vi "SS2 Live_Update Settings & Control.vi"(8 "Error In":errorcluster, 9 "Value":variant, 10 "Sender":string="SS2 DAQ", 11 "CtlRef":refnum<vi>) -> (0 "Error Out":errorcluster, 2 "Control Label":string)   [LabVIEW 2019]
uses:
  SS2 Live_Settings Event.ctl
  SS2 Live_Settings Window Messages.ctl
  Notebook/Notebook.lvlib
  Rich Text Box/Rich Text Box.lvlib
  SS2 Live_Settings List.ctl
  Variant/Variant to Data/Variant to Data.lvlib
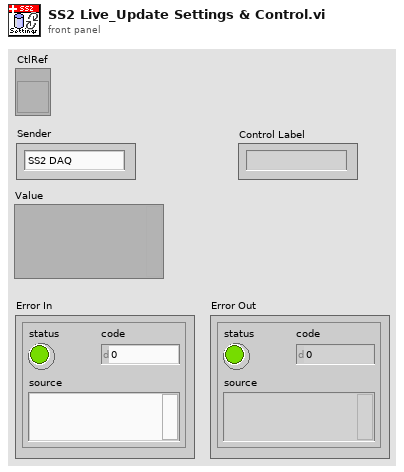
[diagram p1: front panel]
types:
  T1 = typedef "SS2 Live_Settings Event.ctl" = cluster{"Settings Message":T2, "Sender":string, "Control Label":string, "Data":variant}
  T2 = typedef "SS2 Live_Settings Window Messages.ctl" = enum16{"Idle", "Subscribe", "Unsubscribe", "Refresh Parameter", "Refresh All Parameters", "Quit"}
  T3 = typedef "SS2 Live_Settings List.ctl" = enum16{"FPGA:Bitfile Path", "FPGA:Bitfile Version", "Acquisition Parameters:SS2 DAQ Parameters", "Acquisition Parameters:Gate Configuration Array", "Acquisition Parameters:Buffer Size (# Gates)", "File Information:File Information", "File Information:# Datasets in Series", "Image Parameters:Image ROI Information", "Image Parameters:Image Binning Options", "UI Parameters:Histogram Bins Number"}
  T4 = typedef "Rich Text Box.lvlib/Text Formatting.ctl" = cluster{"Font":string, "Text Color":T5, "Text Background Color":T5, "Text Style":enum16{"Regular", "Bold", "Italic", "Underline", "Strikeout"}, "Font Size (Points)":dbl, "Text Alignment":i32}
  T5 = typedef "Rich Text Box.lvlib/Text Colors.ctl" = enum16{"Unchanged", "Black", "Blue", "Gray", "Green", "Red", "White"}
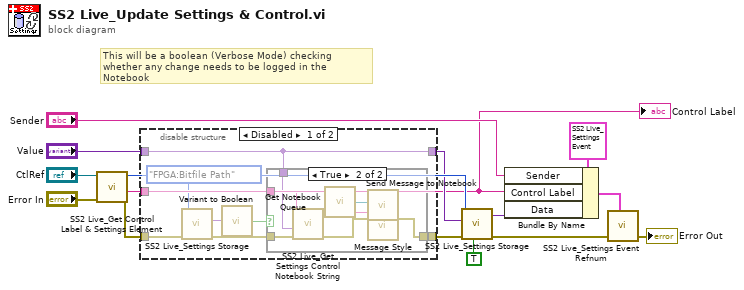
[diagram p0: block diagram]
diagram:
  # "This will be a boolean (Verbose Mode) checking whether any change needs to be logged in the Notebook"
  n1 = call "SS2 Live_Get Control Label & Settings Element.vi"("Error In"="Error In", "CtlRef"="CtlRef") -> ("Error Out"=w5:errorcluster, "Control Label"=w1:string, "Settings Element"=w11:T3)  [unwired: 7 in]
  "Control Label" <- w1
  n2 = disable-structure shown="Disabled" {
    disable-tunnel: w5 -> [w23 w34]
    disable-tunnel: w1 -> [w20 _]
    disable-tunnel: "Value" -> [w16 w33]
    disable-tunnel: [w18 w34] -> w4
    disable-tunnel: [w16 w33] -> w2
    frame Disabled {
      n3 = call "SS2 Live_Settings Storage.vi"("Error In"=w23, "Settings List"=SS2_Live_Settings_List."FPGA:Bitfile Path") -> ("Error Out"=w19:errorcluster, "Variant Data out"=w22:variant)  [unwired: 8 in]
      n4 = call "Variant to Boolean.vi"("Variant"=w22) -> ("Value"=w21:bool)  [unwired: 8 in]
      n5 = case shown="True" w21 {
        tunnel: w20 -> [_ w32]
        tunnel: w16 -> [_ w31]
        tunnel: w19 -> [w24 w30]
        tunnel: [w24 w26] -> w18
        frame False {
        }
        frame True {
          n6 = call "SS2 Live_Get Settings Control Notebook String.vi"("error in (no error)"=w30, "Value"=w31, "Control Label"=w32) -> ("error out"=w27:errorcluster, "Notebook String"=w28:string)  [unwired: 7 in]
          n7 = call "Get Notebook Queue.vi"() -> ("Notebook Queue"=w29:refnum<queue>)  [unwired: 9 in]
          n8 = call "Message Style.vi"() -> ("Message Formatting"=w25:T4)
          n9 = call "Send Message to Notebook.vi"("Notebook Queue"=w29, "Message"=w28, "Error In"=w27, "Text Formatting"=w25) -> ("Error Out"=w26:errorcluster)  [unwired: 15 in]
        }
      }
    }
    frame Enabled {
    }
  }
  n10 = call "SS2 Live_Settings Storage.vi"("Set/Get(F)"=TRUE ("Get(F)/Set"), "Error In"=w4, "Variant Data in"=w2, "Settings List"=w11) -> ("Error Out"=w9:errorcluster, "Variant Data out"=w10:variant)  [unwired: 6 in]
  n11 = Bundle By Name(cluster=T1 {"Settings Message"=enum."Refresh Parameter", "Sender"="", "Control Label"="", "Data"=variant}, "Sender"="Sender", "Control Label"=w1, "Data"=w10) -> (w7:T1)
  n12 = call "SS2 Live_Settings Event Refnum.vi"("Settings Event"=w7, "Error In"=w9) -> ("Error Out"=→"Error Out":errorcluster)  [unwired: 6 in, 1 out]
